vi "Self Correct Rx IQ Offset.vi"() -> ()   [LabVIEW 2021]
uses:
  <vilib>/userDefined/Silver/nirio_resource_slv.ctl
  <vilib>/Utility/error.llb/DialogType.ctl
  <instrlib>/niUsrpRio/Config/v1/Host/Public/EEPROM Data Section.ctl
  <vilib>/Utility/error.llb/Error Cluster From Error Code.vi
  <vilib>/ErrorRing/Error Ring.xnode
  <instrlib>/niUsrpRio/Config/v1/Host/niUsrpRio Config v1 Host.lvlib
panel:
  in  "tuning settle (ms)":u32=100
  in  "reference frequency source":string(combo)="Internal"
  in  "Commit Update to Device?":bool=TRUE
  in  "USRP RIO Device":T1="Select USRP RIO Device"
  # "Select the USRP RIO device on which to run a self-correction of the Rx IQ Offset (LO Feedthrough).  A completed run implies successful update (an error dialog will display if there are errors)."
  # "Specify the time to wait between configuring the frequency\nand measuring the LO Feedthrough."
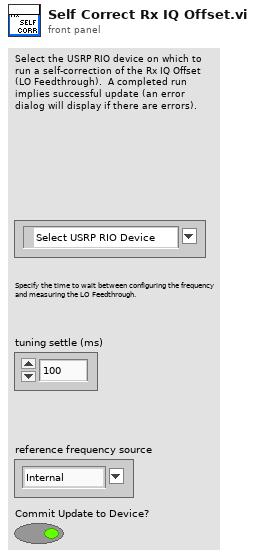
[diagram p1: front panel]
types:
  T1 = typedef "nirio_resource_slv.ctl" = tag
  T2 = typedef "DialogType.ctl" = u16
  T3 = typedef "niUsrpRio Config v1 Host.lvlib/niUsrpRio Session.ctl" = cluster{"FPGA Interface":refnum<k20>, "RIO Interface Number":u32, "Data Clock Rate":u32, "FPGA Data Clock Rate":u32, "Global Settings Register Bus":T4, "Radio 0 Settings Register Bus":T4, "Radio 1 Settings Register Bus":T4, "Radio Settings Bus Semaphore":T5, "DB Queues":T6[], "Characterization Data Valid?":bool, "EEPROM Header":T7, "Device Data Header":T8, "EEPROM Characterization Header":T9, "Characterization Data":T10[], "FPGA Current Version":u32, "FPGA Oldest Compatible Version":u32, "Fixed Logic Current Version":u32, "Fixed Logic Oldest Compatible Version":u32, "FPGA Radio Settings Bus Current Version":u32, "FPGA Radio Settings Bus Oldest Compatible Version":u32, "FPGA Board Config Current Version":u32, "FPGA Board Config Oldest Compatible Version":u32, "Daughterboard Clock Rate":u32, "daughterboard configuration session handles":u64[]}
  T4 = typedef "niInstr Register Bus v0 Host.lvlib/Register Bus Session.ctl" = refnum<queue>
  T5 = typedef "Semaphore RefNum" = refnum<k1>
  T6 = typedef "niUsrpRio Config v1 Host.lvlib/DB Queue Reference.ctl" = refnum<queue>
  T7 = typedef "niUsrpRio Config v1 Host.lvlib/EEPROM Header.ctl" = cluster{"Checksum":u32, "Product Code":u16, "Hardware Current Version":u16, "Hardware Oldest Compatible Version":u16, "EEPROM Map Current Version":u16, "EEPROM Map Oldest Compatible Version":u16, "User Password":string, "Pointer to Factory Header":u32, "Pointer to User Header":u32, "Recommended Interval":u16, "Number of Reserved Bytes":i32, "Number of Daughterboards":u8, "Daughterboard IDs":u16[], "Daughterboard Serial Numbers":string[]}
  T8 = typedef "niUsrpRio Config v1 Host.lvlib/EEPROM Device Data Header.ctl" = cluster{"Checksum":u32, "Number of Channels":u8, "Number of Gain Settings":u16[], "Pointer to Characterization Data":u32[], "Number of Reserved Bytes":i32, "Number of Frequencies":u16[]}
  T9 = typedef "niUsrpRio Config v1 Host.lvlib/EEPROM Characterization Header.ctl" = cluster{"Checksum":u32, "Date":timestamp, "Temperature":sgl, "Misc. Info":string, "Pointer to Device Data Header":u32, "Number of Reserved Bytes":i32}
  T10 = typedef "niUsrpRio Config v1 Host.lvlib/Characterization Data.ctl" = cluster{"Gains[dB]":dbl[], "Frequencies [Hz]":dbl[], "IQ Imbalance Table":T11[], "Measured Gains[dB]":dbl[][]}
  T11 = typedef "niUsrpRio Config v1 Host.lvlib/IQ Imbalance.ctl" = cluster{"Gain Imbalance [linear]":dbl, "Phase Imbalance [radians]":dbl, "Offset":cdb}
  T12 = typedef "niUsrpRio Config v1 Host.lvlib/EEPROM Data Section.ctl" = enum16{"Factory Data", "User Data"}
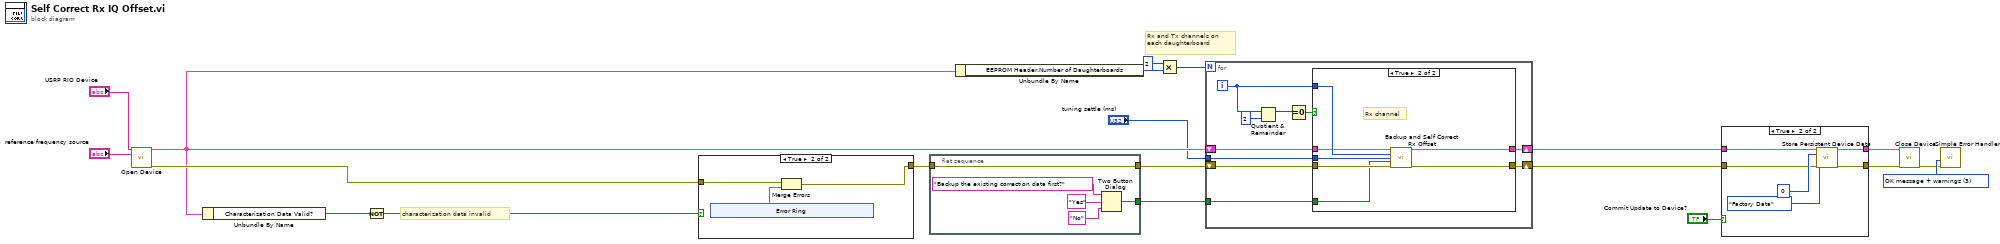
[diagram p0: block diagram]
diagram:
  w20 = T2 3 items=["no dialog", "OK message", "continue or stop message", "OK message + warnings", "continue/stop + warnings"] ("type of dialog (OK msg:1)")
  # "Rx and Tx channels on \neach daughterboard"
  # "characterization data invalid"
  n1 = call "Open Device.vi"("USRP RIO device"="USRP RIO Device", "Reference Frequency Source"="reference frequency source") -> ("niUsrpRio Session (out)"=w6:T3, "error out"=w8:errorcluster)  [unwired: 12 in]
  n2 = Unbundle By Name(w6) -> ("Characterization Data Valid?"=w19:bool)
  n3 = Not(x=w19) -> (.not. x?=w9:bool)
  n4 = case shown="True" w9 {
    tunnel: w8 -> [w21 w24]
    tunnel: [w21 w22] -> w13
    frame False {
    }
    frame True {
      n5 = xnode "Error Ring"() -> ("error out"=w23:errorcluster)
      n6 = Merge Errors(w24, w23) -> (w22:errorcluster)
    }
  }
  n7 = flat-sequence {
    tunnel: w13 -> [w31]
    tunnel: [w31] -> w7
    tunnel: [w30] -> w12
    frame #0 {
      n8 = Two Button Dialog(message="Backup the existing correction data first?", 1:"No" ("F button name (\"Cancel\")"), 2:"Yes" ("T button name (\"OK\")")) -> (T button?=w30:bool)
    }
  }
  n9 = Unbundle By Name(w6) -> ("EEPROM Header.Number of Daughterboards"=w18:u8)
  n10 = Multiply(x=u8 2, y=w18) -> (x*y=w16:u8)
  n11 = for {
    N: w16 -> [_]
    shift-right: [w40] -> w14
    shift-left: w7 -> [w41]
    shift-right: [w37] -> w5
    shift-left: w6 -> [w39]
    tunnel: w12 -> [w36]
    tunnel: "tuning settle (ms)" -> [w35]
    i -> [w38]
    n12 = Quotient & Remainder(x=w38, y=2) -> (x-y*floor(x/y)=w42:i32)  [unwired: 1 out]
    n13 = Equal To 0?(x=w42) -> (x = 0?=w43:bool)
    n14 = case shown="True" w43 {
      tunnel: w41 -> [w45 w51]
      tunnel: [w45 w49] -> w40
      tunnel: w39 -> [w46 w52]
      tunnel: w38 -> [_ w53]
      tunnel: [w46 w50] -> w37
      tunnel: w36 -> [_ w48]
      tunnel: w35 -> [_ w47]
      frame False {
        # "nothing needs to be\ncorrected for Tx"
        # "Tx Channel"
      }
      frame True {
        # "Rx channel"
        n15 = call "Backup and Self Correct Rx Offset.vi"("niUsrpRio session"=w52, "channel to update"=w53, "tuning settle (ms)"=w47, "backup existing data?"=w48, "Error In"=w51) -> ("niUsrpRio session (out)"=w50:T3, "Error Out"=w49:errorcluster)  [unwired: 8 in, 1 out]
      }
    }
  }
  n16 = case shown="True" "Commit Update to Device?" {
    tunnel: w14 -> [w54 w59]
    tunnel: w5 -> [w55 w58]
    tunnel: [w54 w57] -> w4
    tunnel: [w55 w56] -> w3
    frame False {
    }
    frame True {
      n17 = call <instrlib>:"Store Persistent Device Data.vi"("niUsrpRio session"=w58, "offset"=u32 0, "EEPROM Data Section"=EEPROM_Data_Section."Factory Data", "error in"=w59) -> ("niUsrpRio session (out)"=w56:T3, "error out"=w57:errorcluster)  [unwired: 10 in]
    }
  }
  n18 = call "Close Device.vi"("niUsrpRio Session"=w3, "error in"=w4) -> ("error out"=w2:errorcluster)  [unwired: 13 in]
  n19 = call <vilib>:"Simple Error Handler.vi"("type of dialog (OK msg:1)"=w20, "error in (no error)"=w2) -> ()  [unwired: 3 in, 5 out]
